vi "Actor Core.vi"(8 "error in":errorcluster, 11 "Calculator Actor in":refnum<class "Calculator Actor.lvclass">) -> (0 "error out":errorcluster, 3 "Actor out":refnum<class "Actor.lvclass">)   [LabVIEW 2015, in "Calculator Actor.lvclass"]
doc: "(<B>Filename</B>: Actor Framework.lvlib:Actor.lvclass:Actor Core.vi)\n\nReceives messages to the actor, reacts to them, and initiates any error handling that may shut the actor down.\n\nDescendant classes may override this VI to append parallel tasks for the actor to complete while it handles messages. Overrides use the Call Parent Method node."
uses:
  Calculator Actor.lvclass
  <vilib>/ActorFramework/Actor/Actor.lvclass
  Addition Actor/Addition Actor Class/Addition Actor.lvclass
  Multiplication Actor/Multiplication Actor Class/Multiplication Actor.lvclass
  Calculator Actor.lvclass/Calculator Actor.ctl
  <vilib>/ActorFramework/Actor/Actor.lvclass/Actor.ctl
  <vilib>/ActorFramework/Message Enqueuer/Message Enqueuer.lvclass/Message Enqueuer.ctl
  <vilib>/ActorFramework/Message Enqueuer/Init from Existing Queue.vi
  <vilib>/ActorFramework/Message Enqueuer/Enqueue.vi
  <vilib>/ActorFramework/Message Priority Queue/Priority Enqueue.vi
  <vilib>/ActorFramework/Message Enqueuer/Message Enqueuer.lvclass
  <vilib>/ActorFramework/Stop Msg/Stop Msg.lvclass
  Addition Actor/Addition Acotr Messages/Addition Request Msg/Addition Request Msg.lvclass
panel:
  in  "Calculate":bool
  out "Result - Multiplication":dbl
  out "Result - Addition":dbl
  in  "Number 2":dbl
  in  "Number 1":dbl
  in  "stop":bool
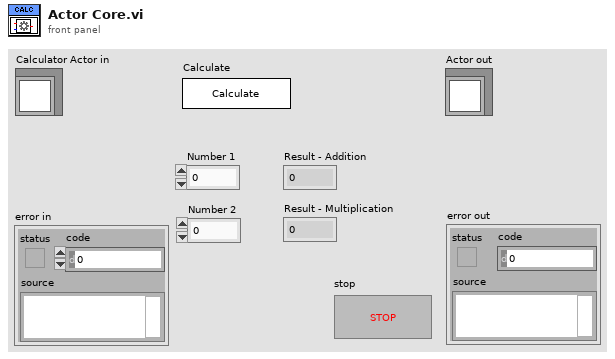
[diagram p1: front panel]
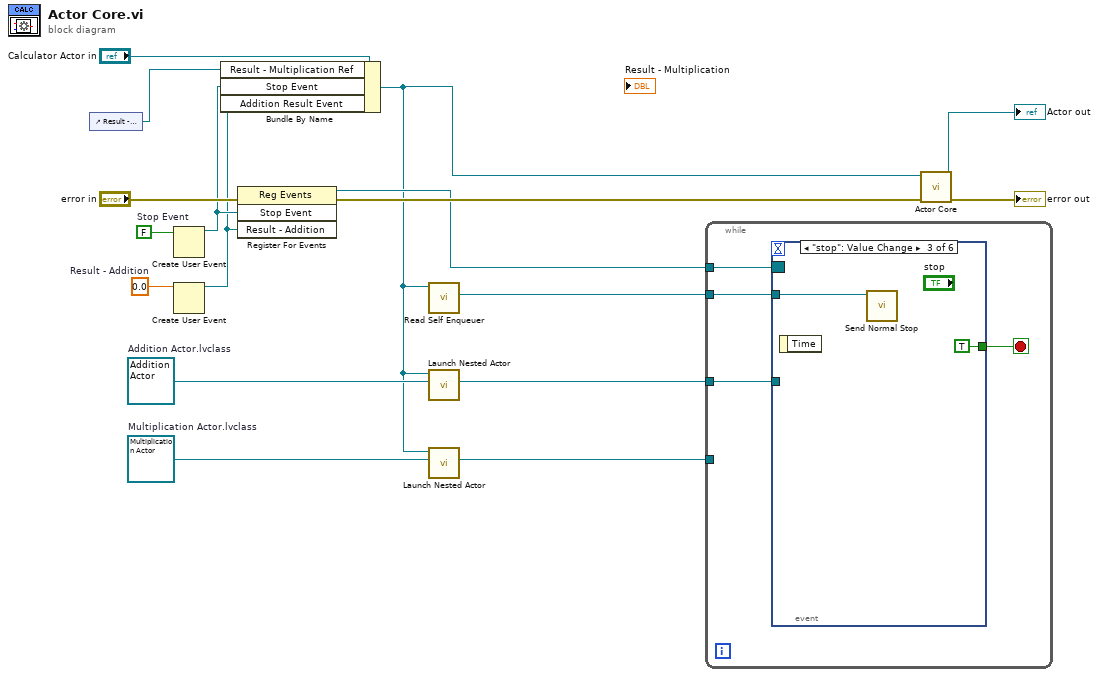
[diagram p0: block diagram]
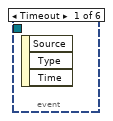
[diagram p2: hidden frame]
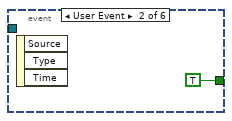
[diagram p3: hidden frame]
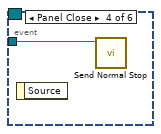
[diagram p4: hidden frame]
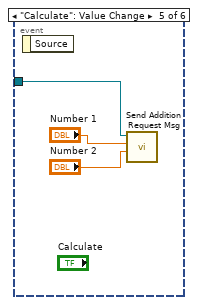
[diagram p5: hidden frame]
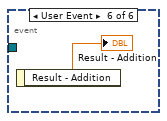
[diagram p6: hidden frame]
diagram:
  w3 = 0.0  # Result - Addition
  w7 = refnum<class "Multiplication Actor.lvclass"> refnum  # Multiplication Actor.lvclass
  w8 = refnum<class "Addition Actor.lvclass"> refnum  # Addition Actor.lvclass
  w13 = FALSE  # Stop Event
  n1 = control-ref of="Result - Multiplication"() -> (w1:refnum<vi>)
  n2 = Create User Event(user event datatype=w13) -> (user event=w10:refnum<user-event>)  [unwired: 1 in, 1 out]
  n3 = Create User Event(user event datatype=w3) -> (user event=w2:refnum<user-event>)  [unwired: 1 in, 1 out]
  n4 = Bundle By Name(cluster="Calculator Actor in", "Result - Multiplication Ref"=w1, "Stop Event"=w10, "Addition Result Event"=w2) -> (w6:refnum<class "Calculator Actor.lvclass">)
  n5 = register-events(error in="error in", w10, w2) -> (reference out=w12:refnum<event-registration>, error out=w14:errorcluster)  [unwired: 1 in]
  n6 = call <vilib>:"Read Self Enqueuer.vi"("Actor"=w6) -> ("Self Enqueuer"=w9:refnum<class "Message Enqueuer.lvclass">)  [unwired: 10 in]
  n7 = call <vilib>:"Launch Nested Actor.vi"("Nested Actor"=w8, "Caller Actor in"=w6) -> ("Nested Actor's Enqueuer"=w5:refnum<class "Message Enqueuer.lvclass">)  [unwired: 7 in, 2 out]
  n8 = call <vilib>:"Launch Nested Actor.vi"("Nested Actor"=w7, "Caller Actor in"=w6) -> ("Nested Actor's Enqueuer"=w4:refnum<class "Message Enqueuer.lvclass">)  [unwired: 7 in, 2 out]
  n9 = while {
    tunnel: w12 -> [w21]
    tunnel: w9 -> [w19]
    tunnel: w5 -> [w18]
    tunnel: w4 -> [_]
    stop <- w20 stop-if-true
    n10 = event shown="[2] \"stop\": Value Change" {
      selector: w21 -> [_ _ _ _ _ _]
      dyn-events: _ -> [_ _ _ _ _ _]
      timeout: _ -> [_ _ _ _ _ _]
      tunnel: [_ TRUE TRUE _ _ _] -> w20
      tunnel: w19 -> [_ _ w24 w25 _ _]
      tunnel: w18 -> [_ _ _ _ w26 _]
      event Timeout {
        n11 = event-data() -> ()  [unwired: 1 in, 3 out]
      }
      event User Event {
        n12 = event-data() -> ()  [unwired: 1 in, 3 out]
      }
      event "stop": Value Change {
        n13 = event-data() -> ()  [unwired: 1 in, 1 out]
        n14 = call <vilib>:"Send Normal Stop.vi"("Message Enqueuer"=w24) -> ()  [unwired: 10 in, 1 out]
      }
      event Panel Close {
        n15 = event-data() -> ()  [unwired: 1 in, 1 out]
        n16 = call <vilib>:"Send Normal Stop.vi"("Message Enqueuer"=w25) -> ()  [unwired: 10 in, 1 out]
      }
      event "Calculate": Value Change {
        n17 = event-data() -> ()  [unwired: 1 in, 1 out]
        n18 = call "Send Addition Request Msg.vi"("Number2"="Number 2", "Number1"="Number 1", "Message Enqueuer in"=w26) -> ()  [unwired: 7 in, 2 out]
      }
      event User Event {
        n19 = event-data() -> ("Result - Addition"=→"Result - Addition":dbl)  [unwired: 1 in]
      }
    }
  }
  n20 = call-parent "Actor Core.vi"("error in"=w14, "Actor in"=w6) -> ("error out"=→"error out":errorcluster, "Actor out"=→"Actor out":refnum<class "Actor.lvclass">)  [unwired: 8 in]
